vi "myRIO__TCP_write.vi"(8 "input_error":errorcluster, 10 "input_packet":string, 11 "input_hTCP":refnum<k5>) -> (0 "output_error":errorcluster, 2 "output_I_write":bool, 3 "output_hTCP":refnum<k5>)   [LabVIEW 2014]
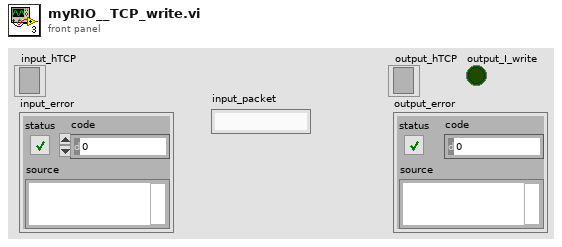
[diagram p1: front panel]
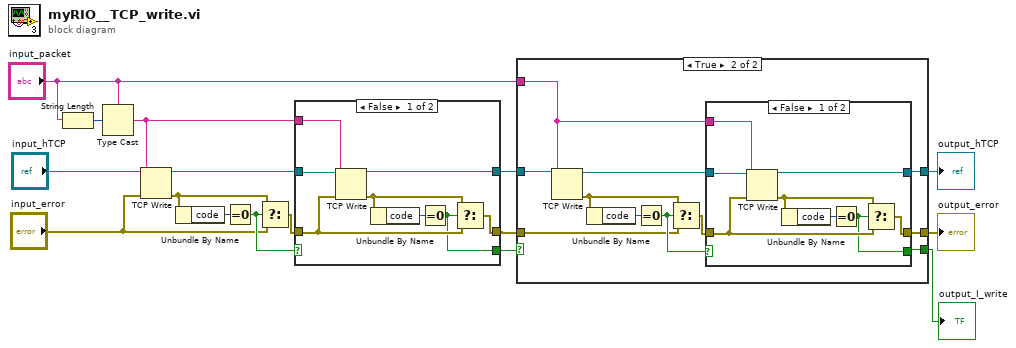
[diagram p0: block diagram]
diagram:
  n1 = String Length(string="input_packet") -> (length=w9:i32)
  n2 = Type Cast(type="input_packet", x=w9) -> (*(type *) &x=w8:string)
  n3 = TCP Write(connection ID="input_hTCP", data in=w8, error in (no error)="input_error") -> (connection ID out=w12:refnum<k5>, error out=w14:errorcluster)  [unwired: 2 out]
  n4 = Unbundle By Name(w14) -> ("code"=w15:i32)
  n5 = Equal To 0?(x=w15) -> (x = 0?=w13:bool)
  n6 = Select(t=w14, s=w13, f="input_error") -> (s? t:f=w10:errorcluster)
  n7 = case shown="False" w13 {
    selector: w13 -> [_ w25]
    tunnel: w12 -> [w22 w26]
    tunnel: w10 -> [w20 w27]
    tunnel: [w18 w27] -> w6
    tunnel: [w19 w26] -> w5
    tunnel: w8 -> [w21 _]
    tunnel: [w17 w25] -> w7
    frame False {
      n8 = TCP Write(connection ID=w22, data in=w21, error in (no error)=w20) -> (connection ID out=w19:refnum<k5>, error out=w23:errorcluster)  [unwired: 2 out]
      n9 = Unbundle By Name(w23) -> ("code"=w24:i32)
      n10 = Equal To 0?(x=w24) -> (x = 0?=w17:bool)
      n11 = Select(t=w23, s=w17, f=w20) -> (s? t:f=w18:errorcluster)
    }
    frame True {
    }
  }
  n12 = case shown="True" w7 {
    selector: w7 -> [w28 _]
    tunnel: w6 -> [w29 w36]
    tunnel: w5 -> [w30 w35]
    tunnel: "input_packet" -> [_ w34]
    tunnel: [w30 w31] -> w3
    tunnel: [w29 w32] -> w2
    tunnel: [w28 w33] -> w1
    frame False {
    }
    frame True {
      n13 = TCP Write(connection ID=w35, data in=w34) -> (connection ID out=w38:refnum<k5>, error out=w40:errorcluster)  [unwired: 1 in, 2 out]
      n14 = Unbundle By Name(w40) -> ("code"=w41:i32)
      n15 = Equal To 0?(x=w41) -> (x = 0?=w39:bool)
      n16 = Select(t=w40, s=w39, f=w36) -> (s? t:f=w37:errorcluster)
      n17 = case shown="False" w39 {
        selector: w39 -> [_ w50]
        tunnel: w38 -> [w47 w51]
        tunnel: w37 -> [w45 w52]
        tunnel: [w43 w52] -> w32
        tunnel: [w44 w51] -> w31
        tunnel: w34 -> [w46 _]
        tunnel: [w42 w50] -> w33
        frame False {
          n18 = TCP Write(connection ID=w47, data in=w46, error in (no error)=w45) -> (connection ID out=w44:refnum<k5>, error out=w48:errorcluster)  [unwired: 2 out]
          n19 = Unbundle By Name(w48) -> ("code"=w49:i32)
          n20 = Equal To 0?(x=w49) -> (x = 0?=w42:bool)
          n21 = Select(t=w48, s=w42, f=w45) -> (s? t:f=w43:errorcluster)
        }
        frame True {
        }
      }
    }
  }
  "output_hTCP" <- w3
  "output_error" <- w2
  "output_I_write" <- w1
